vi "S11 to Z frequency.vi"(8 "Error In":errorcluster, 9 "S11":T1 {"Z" format="%#_4g"}, 10 "Ref. Z [Ohm]":cdb=50.0+0.0i) -> (0 "Error Out":errorcluster, 1 "Z":T1 {"Z" format="%#_4g"})   [LabVIEW 2016]
uses:
  Trace (cplx).ctl
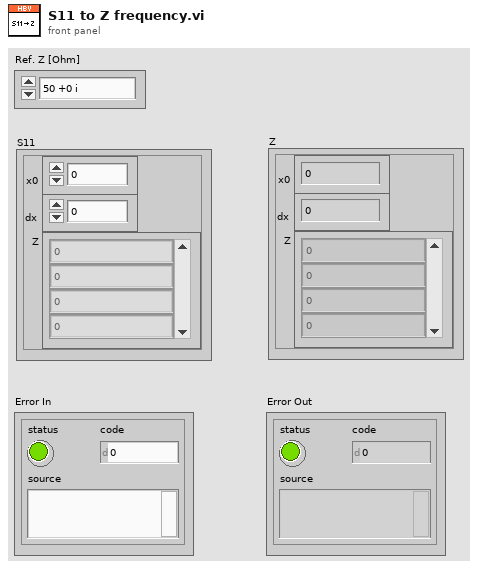
[diagram p1: front panel]
types:
  T1 = typedef "Trace (cplx).ctl" = cluster{"x0":dbl, "dx":dbl, "Z":cdb[]}
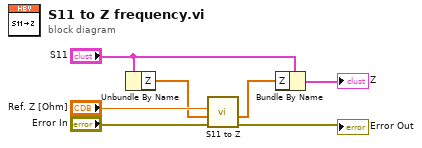
[diagram p0: block diagram]
diagram:
  n1 = Unbundle By Name("S11") -> ("Z"=w5:cdb[])
  n2 = call "S11 to Z.vi"("Error In"="Error In", "S11"=w5, "Ref. Z [Ohm]"="Ref. Z [Ohm]") -> ("Error Out"=→"Error Out":errorcluster, "Z [Ohm]"=w7:cdb[])  [unwired: 7 in]
  n3 = Bundle By Name(cluster="S11", "Z"=w7) -> (→"Z":T1)
